vi "UART кон. авт. тест.vi"() -> ()   [LabVIEW 2012]
doc: "Use this template to build a standard state machine design pattern. Each state executes code and determines which state to transition to. Contrast this design pattern with the User Interface Event Handler pattern, in which code executes in response to user actions. Contrast this design pattern also with the Queued Message Handler pattern, in which each message handling code can queue zero or more new messages."
uses:
  StateMachineStates 3.ctl
  <vilib>/Utility/error.llb/DialogType.ctl
  <vilib>/Instr/_visa.llb/VISA Configure Serial Port (Instr).vi
panel:
  out "Reading":bool
  out "bytes red":u32
  out "read":string
  out "Bytes at Serial Port":u32
  out "err":string=" INSTRUCTIONS:\r\rNormal Use:  When using subVIs that incorporate the error in/error out (or error I/O) structure, place this handler where you want to inform the user of an error, typically at the end of the I/O data path, as the last action of the program.  If the error in error? is ERROR, the handler creates a message describing the error and its source.  If the type of dialog = 1 (default), the message is displayed to the user, who can only acknowedge it.  If the type = 2, the user can acknowledge the message or abort execution; aborting a program with active I/O is not recommended.  If the type = 0, no message is displayed; this is used to process the error programmatically, and the error out cluster elements are wired to individual terminals for that reason.  \r\rOther Use:\n\r\nlocal testing.  To test the error code of a subVI or function that does not have the error I/O structure, you can wire its error code and a source string to the local error code and error source inputs.  If error in error? indicates no error and error code is not equal to 0, the local code and source are substituted for the error in values, and error? is set TRUE (ERROR)."
  in  "stop":bool
  in  "VISA resource name":refnum<visa-resource-name>
  in  "baud rate (9600)":u32=9600
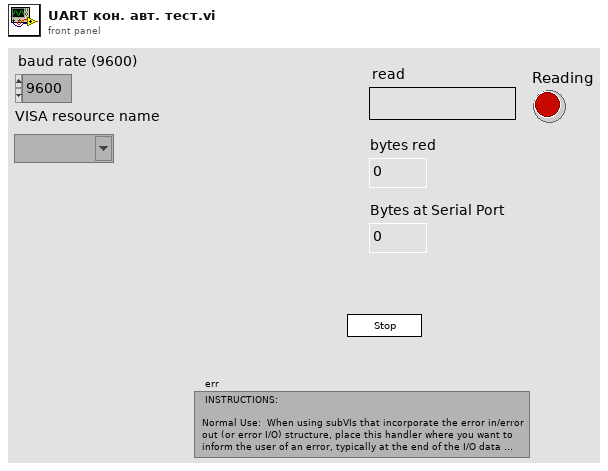
[diagram p1: front panel]
types:
  T1 = typedef "StateMachineStates 3.ctl" = enum16{"Initialize", "read port", "Stop"}
  T2 = typedef "DialogType.ctl" = u16
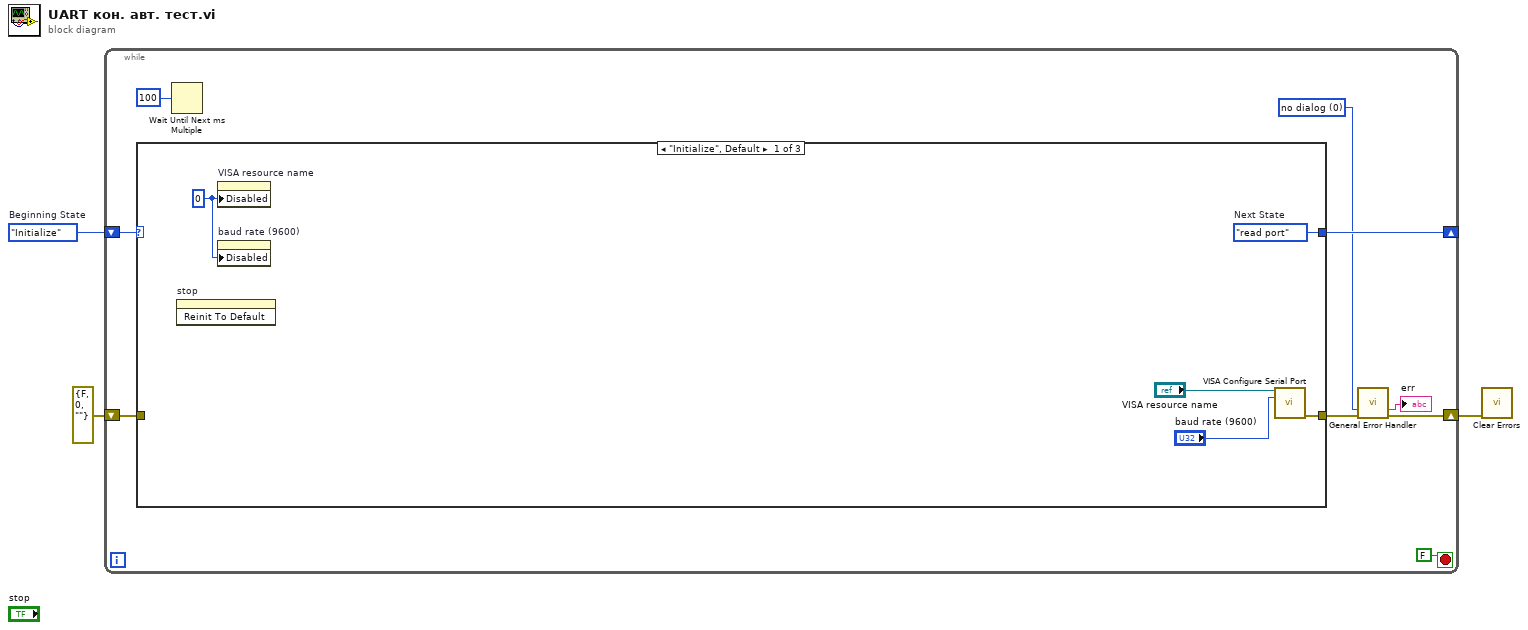
[diagram p0: block diagram]
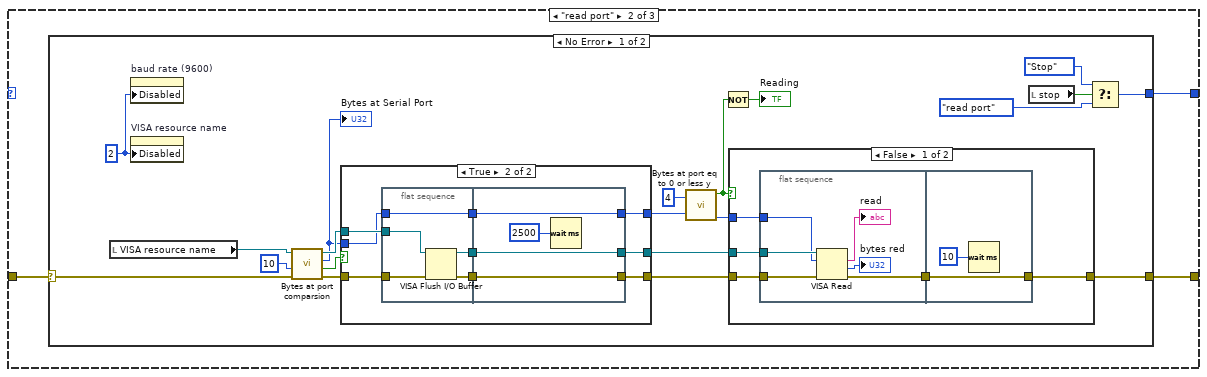
[diagram p2: hidden frame]
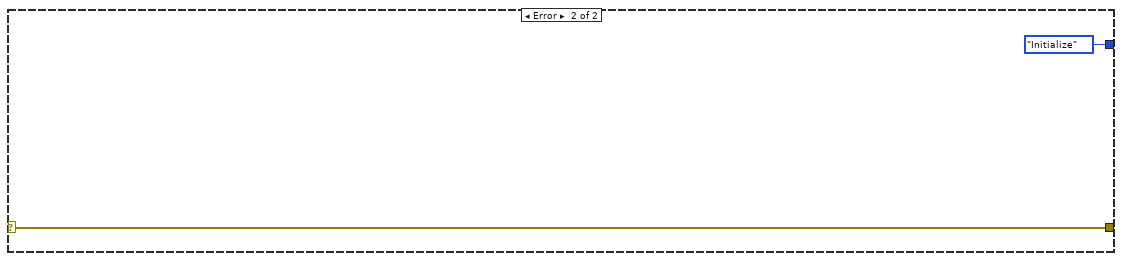
[diagram p5: hidden frame]
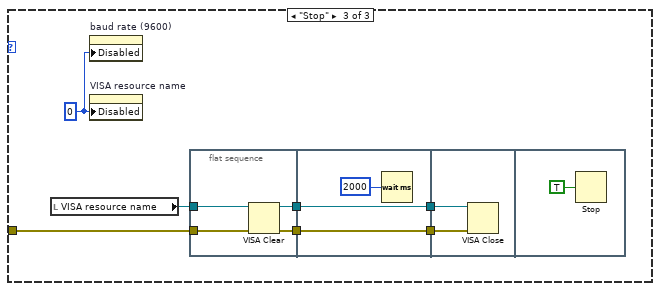
[diagram p6: hidden frame]
diagram:
  w3 = StateMachineStates_3."Initialize"  # Beginning State
  n1 = while {
    shift-right: [w11] -> _
    shift-left: w3 -> [w12]
    shift-right: [w8] -> w1
    shift-left: errorcluster {"status"=FALSE, "code"=0, "source"=""} ("error out") -> [w10]
    stop <- FALSE stop-if-true
    w7 = T2 0 items=["no dialog", "OK message", "continue or stop message", "OK message + warnings", "continue/stop + warnings"] ("type of dialog (OK msg:1)")
    n2 = case shown="\"Initialize\", Default" w12 {
      tunnel: [w17 w18 _] -> w11
      tunnel: [w13 w20 _] -> w9
      tunnel: w10 -> [_ w19 w82]
      frame "Initialize", Default {
        w16 = u8 0 ("Disabled")
        w17 = StateMachineStates_3."read port"  # Next State
        n3 = invoke on="stop" class="Bool (strict)" method="Reinit To Default"() -> ()  [unwired: 3 in, 3 out]
        n4 = property on="VISA resource name" class="VISAName"("Disabled"=w16) -> ()  [unwired: 2 in, 2 out]
        n5 = property on="baud rate (9600)" class="DigNum (strict)"("Disabled"=w16) -> ()  [unwired: 2 in, 2 out]
        n6 = call-poly "VISA Configure Serial Port"("VISA resource name"="VISA resource name", "baud rate (9600)"="baud rate (9600)") -> ("error out"=w13:errorcluster)  [unwired: 4 in, 9 out]
      }
      frame "read port" {
        n7 = case shown="No Error" w19 {
          selector: w19 -> [w34 w77]
          tunnel: [w28 w77] -> w20
          tunnel: [w37 StateMachineStates_3."Initialize" ("Next State")] -> w18
          frame No Error {
            w40 = u8 2 ("Disabled")
            n8 = local read "VISA resource name"() -> (w35:refnum<visa-resource-name>)
            n9 = property on="baud rate (9600)" class="DigNum (strict)"("Disabled"=w40) -> ()  [unwired: 2 in, 2 out]
            n10 = property on="VISA resource name" class="VISAName"("Disabled"=w40) -> ()  [unwired: 2 in, 2 out]
            n11 = call "Bytes at port comparsion.vi"("error in (no error)"=w34, "x"=u32 10, "VISA Refnum in"=w35) -> ("error out"=w30:errorcluster, "bytes more then X ?"=w33:bool, "Bytes at Port"=w27:u32, "VISA Refnum out"=w29:refnum<visa-resource-name>)  [unwired: 5 in]
            "Bytes at Serial Port" <- w27
            n12 = case shown="True" w33 {
              tunnel: [w43 w52] -> w32
              tunnel: [w42 w48] -> w31
              tunnel: w30 -> [w43 w50]
              tunnel: w29 -> [w42 w49]
              tunnel: w27 -> [w41 w45]
              tunnel: [w41 w44] -> w23
              frame False {
              }
              frame True {
                n13 = flat-sequence {
                  tunnel: [w57] -> w51
                  tunnel: w50 -> [w56]
                  tunnel: w49 -> [w55]
                  tunnel: [w54] -> w47
                  tunnel: [w53] -> w46
                  tunnel: w45 -> [w53]
                  tunnel: [w61] -> w52
                  tunnel: w51 -> [w61]
                  tunnel: [w59] -> w48
                  tunnel: w47 -> [w59]
                  tunnel: w46 -> [w58]
                  tunnel: [w58] -> w44
                  frame #0 {
                    n14 = VISA Flush I/O Buffer(VISA resource name=w55, error in (no error)=w56) -> (VISA resource name out=w54:refnum<visa-resource-name>, error out=w57:errorcluster)  [unwired: 1 in]
                  }
                  frame #1 {
                    n15 = Wait (ms)(milliseconds to wait=u32 2500) -> ()  [unwired: 1 out]
                  }
                }
              }
            }
            n16 = call "Bytes at port eq to 0 or less y.vi"("y"=u32 4, "Bytes at Port"=w23) -> ("Bytes at port = 0 or less y"=w24:bool, "Bytes at Port out"=w21:u32)  [unwired: 4 in]
            n17 = Not(x=w24) -> (.not. x?=→"Reading":bool)
            n18 = case shown="False" w24 {
              tunnel: [w66 w75] -> w28
              tunnel: w32 -> [w65 w75]
              tunnel: w31 -> [w64 _]
              tunnel: w21 -> [w62 _]
              frame False {
                n19 = flat-sequence {
                  tunnel: w65 -> [w71]
                  tunnel: w64 -> [w68]
                  tunnel: [w72] -> w63
                  tunnel: w62 -> [w67]
                  tunnel: [w74] -> w66
                  tunnel: w63 -> [w74]
                  frame #0 {
                    n20 = VISA Read(VISA resource name=w68, byte count=w67, error in (no error)=w71) -> (read buffer=→"read":string, return count=→"bytes red":u32, error out=w72:errorcluster)  [unwired: 1 out]
                  }
                  frame #1 {
                    n21 = Wait (ms)(milliseconds to wait=u32 10) -> ()  [unwired: 1 out]
                  }
                }
              }
              frame True {
              }
            }
            n22 = local read "stop"() -> (w36:bool)
            n23 = Select(t=StateMachineStates_3."Stop" ("Next State"), s=w36, f=StateMachineStates_3."read port" ("Next State")) -> (s? t:f=w37:T1)
          }
          frame Error {
          }
        }
      }
      frame "Stop" {
        w84 = u8 0 ("Disabled")
        n24 = local read "VISA resource name"() -> (w81:refnum<visa-resource-name>)
        n25 = property on="baud rate (9600)" class="DigNum (strict)"("Disabled"=w84) -> ()  [unwired: 2 in, 2 out]
        n26 = property on="VISA resource name" class="VISAName"("Disabled"=w84) -> ()  [unwired: 2 in, 2 out]
        n27 = flat-sequence {
          tunnel: [w88] -> w83
          tunnel: w82 -> [w87]
          tunnel: w81 -> [w86]
          tunnel: [w85] -> w80
          tunnel: w83 -> [w90]
          tunnel: w80 -> [w89]
          tunnel: [w90] -> w79
          tunnel: [w89] -> w78
          tunnel: w79 -> [w93]
          tunnel: w78 -> [w92]
          frame #0 {
            n28 = VISA Clear(VISA resource name=w86, error in (no error)=w87) -> (VISA resource name out=w85:refnum<visa-resource-name>, error out=w88:errorcluster)
          }
          frame #1 {
            n29 = Wait (ms)(milliseconds to wait=u32 2000) -> ()  [unwired: 1 out]
          }
          frame #2 {
            n30 = VISA Close(VISA resource name=w92, error in (no error)=w93) -> ()  [unwired: 1 out]
          }
          frame #3 {
            n31 = Stop(stop? (T)=TRUE ("Stop")) -> ()
          }
        }
      }
    }
    n32 = Wait Until Next ms Multiple(millisecond multiple=u32 100 ("milliseconds to wait")) -> ()  [unwired: 1 out]
    n33 = call <vilib>:"General Error Handler.vi"("type of dialog (OK msg:1)"=w7, "error in (no error)"=w9) -> ("message"=→"err":string, "error out"=w8:errorcluster)  [unwired: 12 out]
  }
  n34 = call <vilib>:"Clear Errors.vi"("error in (no error)"=w1) -> ()  [unwired: 6 in, 1 out]
